vi "NanotecSMCPD.emergency off.vi"(0 "i ref in":refnum<vi>, 3 "ms timeout (10000)":i32=10000, 5 "error in (no error)":errorcluster) -> (14 "i ref out":refnum<vi>, 17 "timed out":bool, 19 "error out":errorcluster)   [LabVIEW 2014, in "NanotecSMCPD.lvlib"]
doc: "Performs an emergency off, by aborting the movements of all axes."
uses:
  NanotecSMCPD.lvlib
  CS_Core/CSSystem/CoreDefs/CoreDefs.error_type.ctl
  CS_Core/CSSystem/CoreDefs/CoreDefs.error_severity.ctl
  CS_Core/CSApplicationBaseClasses/MotorBase/MotorBase.lvlib
  CS_Core/CSSystem/CoreLib/CoreLib.lvlib
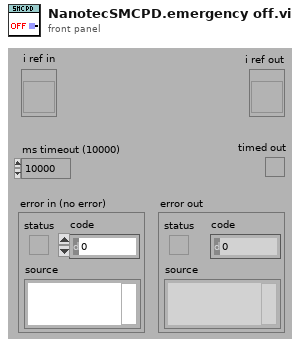
[diagram p1: front panel]
types:
  T1 = typedef "CoreDefs.error_severity.ctl" = enum16{"undefined", "information", "warning", "error", "fatal"}
  T2 = typedef "CoreDefs.error_type.ctl" = enum16{"no error", "can't load process", "can't unload process", "process does not exist", "can't install process", "can't remove process", "unknown function", "time out", "can't execute function", "duplicate queue name", "super not found", "caller queue invalid", "can't ping process", "unknown error", "VISA Error", "VISA timeout", "GPIB timeout", "GPIB error", "communication error", "data type mismatch", "can't read data from OPC server", "can't write data to OPC server", "OET error", "function not implemented", "process already exists", "invalid Shared Variable name", "error writing Shared Variable", "error reading Shared Variable", "invalid client name", "corrupt database", "unknown class", "call not authorized", "parameter out of range", "OET timeout: can't get data to modify", "invalid queue name", "requested operation incompatible with current state", "event undefined", "event disabled", "state undefined", "caller is not a friend", "EventBuilder: bad eventID", "EventBuilder: no DAQ devices", "a thread must not stop itself", "UNUSED ELEMENT4", "DiscArchiver: eventData incomplete", "DiscArchiver: eventData does not belong to run", "DiscArchiver: can't open file", "DiscArchiver: can't write to file", "DiscArchiver: available disc space low", "can't acquire semaphore", "error reading data from database", "notifier object is not existing", "can't register process", "can't unregister process", "illegal event type", "object disabled", "object already exists", "can't change state", "Instrument not found", "no connection to remote node", "invalid reference", "N/A", "UNUSED ELEMENT 1", "element not found", "illegal TCP/IP connection detected", "object does not exist", "invalid access ID", "unknown CS system", "invalid privilige", "unsupported data type", "unsupported server type", "IO server already exists", "Shared Variable already exists"}
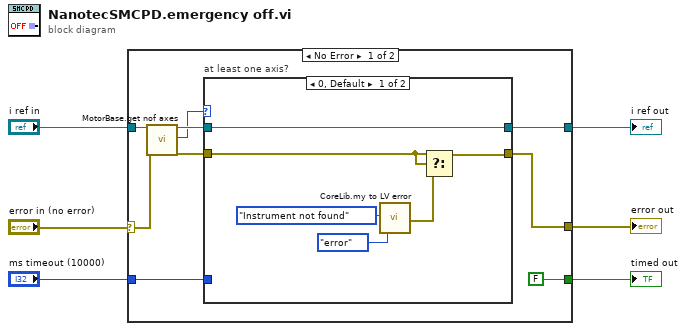
[diagram p0: block diagram]
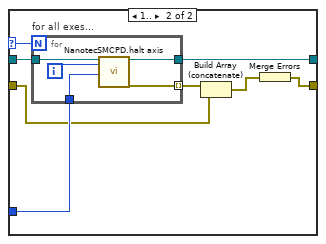
[diagram p2: hidden frame]
diagram:
  n1 = case shown="No Error" "error in (no error)" {
    selector: "error in (no error)" -> [w13 w35]
    tunnel: "i ref in" -> [w15 w36]
    tunnel: [w9 w36] -> w5
    tunnel: [w8 w35] -> w4
    tunnel: "ms timeout (10000)" -> [w12 _]
    tunnel: [FALSE _] -> w1
    frame No Error {
      n2 = call "MotorBase.get nof axes.vi"("i ref in"=w15, "error in (no error)"=w13) -> ("i ref out"=w14:refnum<vi>, "nOfAxis"=w10:i32, "error out"=w11:errorcluster)  [unwired: 15 in]
      n3 = case "at least one axis?" shown="0, Default" w10 {
        selector: w10 -> [_ w29]
        tunnel: w14 -> [w21 w28]
        tunnel: w12 -> [_ w27]
        tunnel: w11 -> [w17 w25]
        tunnel: [w21 w24] -> w9
        tunnel: [w16 w22] -> w8
        frame 0, Default {
          n4 = call "CoreLib.my to LV error.vi"("ErrorTypes"=CoreDefs.error_type."Instrument not found", "severityLevel"=CoreDefs.error_severity."error") -> ("myErrorCluster"=w18:errorcluster)  [unwired: 16 in, 1 out]
          n5 = Select(t=w17, s=w17, f=w18) -> (s? t:f=w16:errorcluster)
        }
        frame 1.. {
          n6 = for "for all exes..." {
            N: w29 -> [_]
            tunnel: w28 -> [w34]
            tunnel: w27 -> [w32]
            tunnel: [w31] -> w24
            tunnel: [w30] -> w26 mode=indexing
            i -> [w33]
            n7 = call "NanotecSMCPD.halt axis.vi"("i ref in"=w34, "axis"=w33, "ms timeout (10000)"=w32) -> ("i ref out"=w31:refnum<vi>, "error out"=w30:errorcluster)  [unwired: 14 in, 1 out]
          }
          n8 = Build Array (concatenate)(w26, w25) -> (w23:errorcluster[])
          n9 = Merge Errors(w23) -> (w22:errorcluster)
        }
      }
    }
    frame Error {
    }
  }
  "error out" <- w4
  "i ref out" <- w5
  "timed out" <- w1
